vi "Default Entry Value--U32.vi"(10 "Theme Control Property":T1, 11 "Window Element":T2) -> (3 "Default Value As U32":u32)   [LabVIEW 2021, in "Appearance Actor.lvlib" / "Generic Theme.lvclass"]
doc: "For a given <B>Window Element</B> and <B>Theme Control Property</B> pair (Theme Entry), returns the corresponding default value for String entries."
uses:
  Generic Theme.lvclass
  Typedefs/Window Element--enum.ctl
  Typedefs/Theme Control Property--enum.ctl
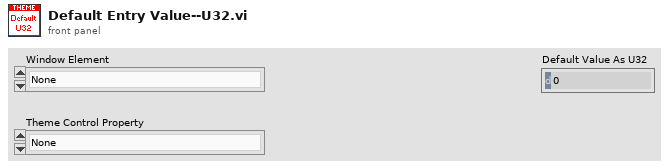
[diagram p1: front panel]
types:
  T1 = typedef "Appearance Actor.lvlib/Generic Theme.lvclass/Theme Control Property--enum.ctl" = enum16{"None", "Button.FalseFillColor", "Button.FalseOutlineColor", "Button.FalseToTrueFillColor", "Button.FalseToTrueOutlineColor", "Button.HoverFalseFillColor", "Button.HoverFalseOutlineColor", "Button.HoverTrueFillColor", "Button.HoverTrueOutlineColor", "Button.TrueFillColor", "Button.TrueOutlineColor", "Button.TrueToFalseFillColor", "Button.TrueToFalseOutlineColor", "CloseButton.FalseFillColor", "CloseButton.FalseOutlineColor", "CloseButton.FalseToTrueFillColor", "CloseButton.FalseToTrueOutlineColor", "CloseButton.HoverFalseFillColor", "CloseButton.HoverFalseOutlineColor", "CloseButton.HoverTrueFillColor", "CloseButton.HoverTrueOutlineColor", "CloseButton.TrueFillColor", "CloseButton.TrueOutlineColor", "CloseButton.TrueToFalseFillColor", "CloseButton.TrueToFalseOutlineColor", "Pane.Color", "Splitter.FillColor", "Splitter.OutlineColor", "Splitter.Size", "Title.Font.Color", "Title.Font.Family", "Title.Font.Size", "Title.Font.Style"}
  T2 = typedef "Appearance Actor.lvlib/Generic Theme.lvclass/Window Element--enum.ctl" = enum16{"None", "TB", "SM", "BP", "SB"}
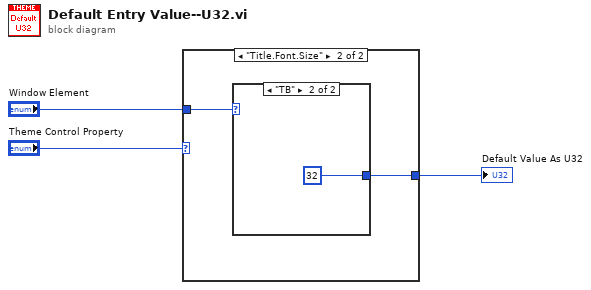
[diagram p0: block diagram]
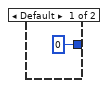
[diagram p2: hidden frame]
diagram:
  n1 = case shown="\"Title.Font.Size\"" "Theme Control Property" {
    tunnel: [u32 0 ("Default Value") w6] -> w3
    tunnel: "Window Element" -> [_ w5]
    frame Default {
    }
    frame "Title.Font.Size" {
      n2 = case shown="\"TB\"" w5 {
        tunnel: [_ u32 32 ("Default Value")] -> w6
        frame Default {
        }
        frame "TB" {
        }
      }
    }
  }
  "Default Value As U32" <- w3
